vi "Waveform Gen.vi"(9 "Inputs":T1={"Frequency1"=2000.0, "Bit Duration in ms"=0.05, "Frequency2"=4000.0, "Amplitude Scale"=1.0, "Sampling Rate"=50000} {"Frequency2" format="%#_13g"; "Frequency1" format="%#_13g"}, 11 "Message String":string="A") -> (0 "Total Message Duration":dbl=0.4, 1 "Waveform Array":u16[](array[numeric]), 2 "No. of Points":u64=20000, 4 "Actual Message Duration":dbl=0.4, 5 "Waveform Graph":u16[](graph))   [LabVIEW 2021]
uses:
  <vilib>/Analysis/NI_AALPro.lvlib
panel:
  out "length":i32
  out "Array":bool[](array[boolean])
  out "Number of characters possible":dbl
  out "Memory exceeded":bool
  out "size(s)":i32
  out "Bit Stram Indicator":u16
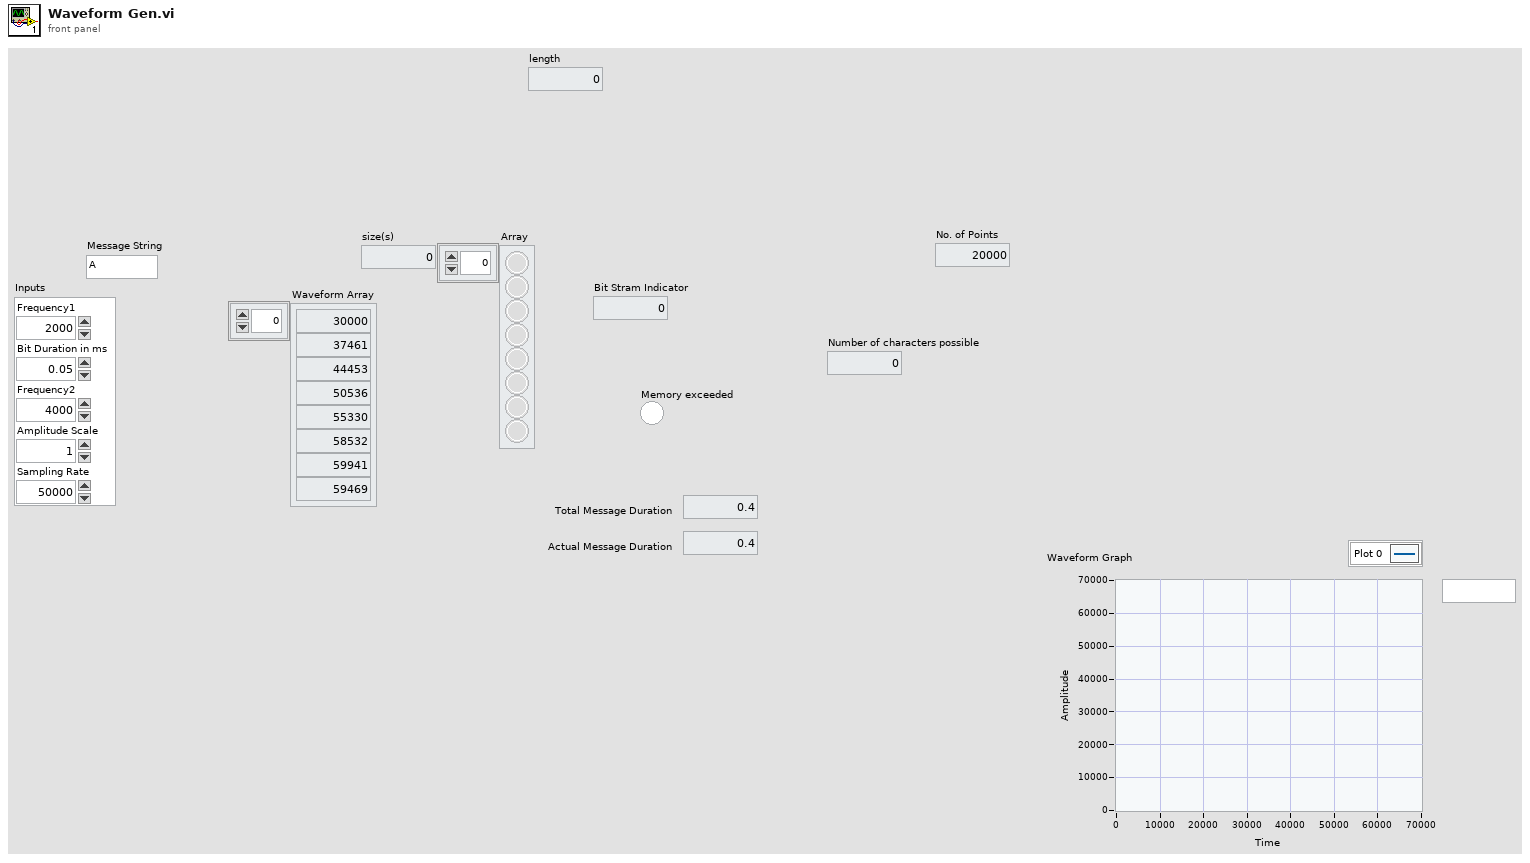
[diagram p1: front panel]
types:
  T1 = cluster{"Frequency1":dbl, "Bit Duration in ms":dbl, "Frequency2":dbl, "Amplitude Scale":dbl, "Sampling Rate":u32}
  T2 = enum16{"sine", "cosine", "triangle", "square", "sawtooth", "increasing ramp", "decreasing ramp"}
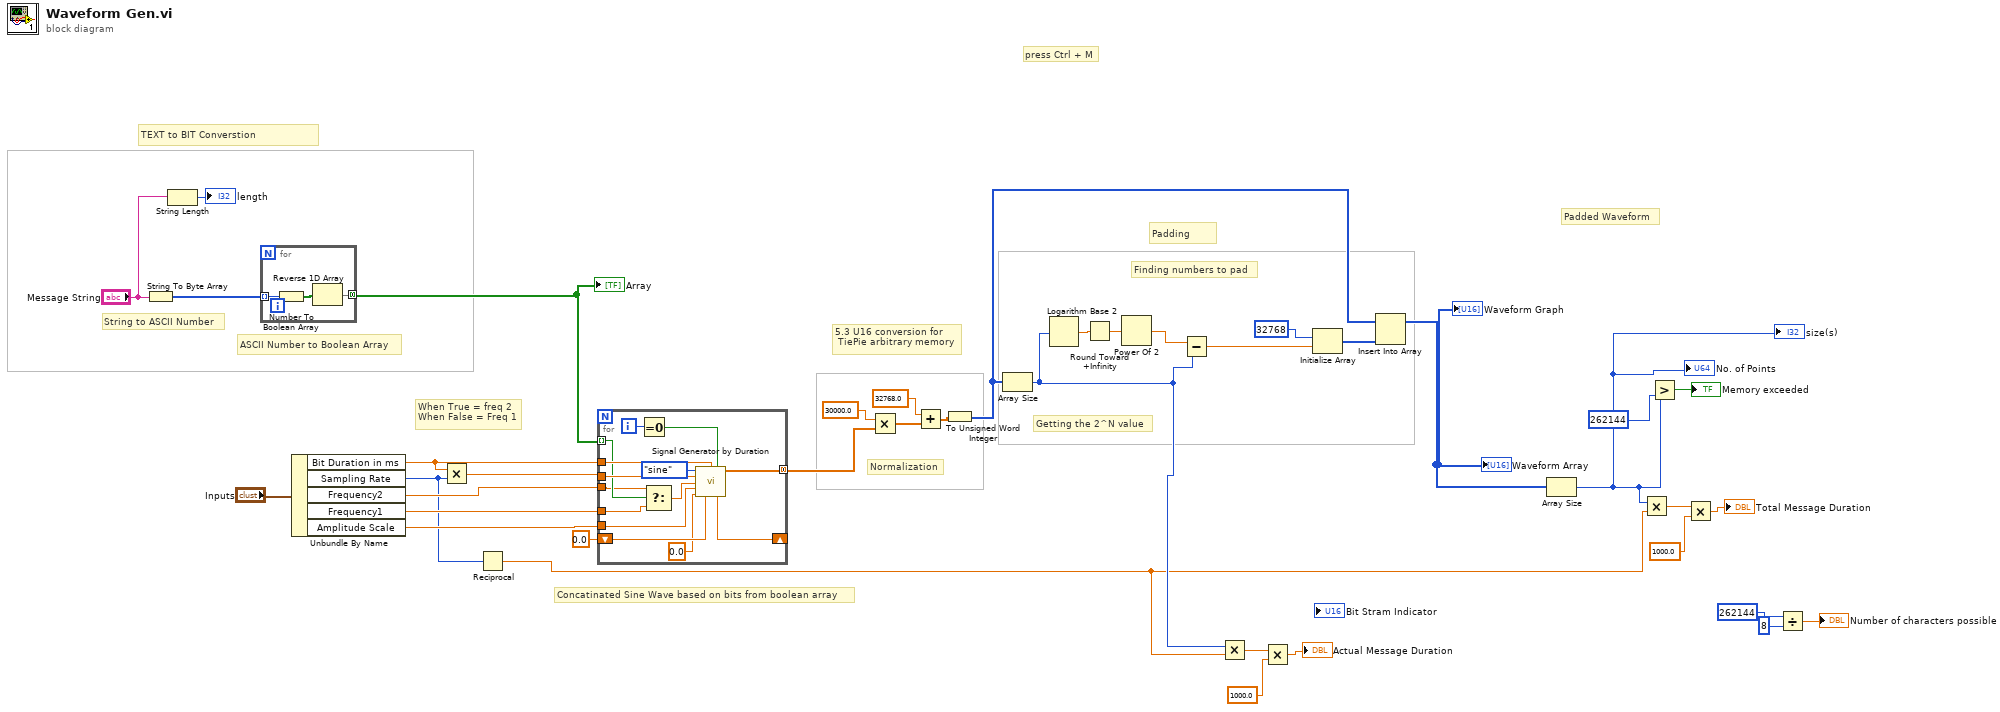
[diagram p0: block diagram]
diagram:
  # "Padding"
  # "5.3 U16 conversion for\n TiePie arbitrary memory"
  # "TEXT to BIT Converstion"
  # "Padded Waveform"
  # "Finding numbers to pad"
  # "Getting the 2^N value"
  # "Normalization"
  # "When True = freq 2\nWhen False = Freq 1"
  # "Concatinated Sine Wave based on bits from boolean array"
  # "ASCII Number to Boolean Array"
  # "String to ASCII Number"
  # "press Ctrl + M"
  n1 = String To Byte Array(string="Message String") -> (unsigned byte array=w39:u8[])
  n2 = String Length(string="Message String") -> (length=→"length":i32)
  n3 = for {
    tunnel: w39 -> [w42] mode=indexing
    tunnel: [w40] -> w38 mode=concatenating
    n4 = Number To Boolean Array(number=w42) -> (Boolean array=w41:bool[])
    n5 = Reverse 1D Array(array=w41) -> (reversed array=w40:bool[])
  }
  "Array" <- w38
  n6 = Unbundle By Name("Inputs") -> ("Bit Duration in ms"=w36:dbl, "Sampling Rate"=w30:u32, "Frequency2"=w34:dbl, "Frequency1"=w33:dbl, "Amplitude Scale"=w31:dbl)
  n7 = Multiply(x=w36, y=w30) -> (x*y=w35:dbl)
  n8 = Reciprocal(x=w30) -> (1/x=w6:dbl)
  n9 = for {
    tunnel: w38 -> [w51] mode=indexing
    tunnel: w36 -> [w54]
    tunnel: w35 -> [w53]
    tunnel: w34 -> [w50]
    tunnel: w33 -> [w49]
    shift-right: [w48] -> _
    shift-left: 0.0 ("phase out") -> [w47]
    tunnel: w31 -> [w44]
    tunnel: [w45] -> w25 mode=concatenating
    i -> [w56]
    n10 = Equal To 0?(x=w56) -> (x = 0?=w55:bool)
    n11 = Select(t=w50, s=w51, f=w49) -> (s? t:f=w52:dbl)
    n12 = call <vilib>:"Signal Generator by Duration.vi"("signal type"=T2."sine", "duration"=w54, "reset phase"=w55, "# of samples"=w53, "frequency"=w52, "amplitude"=w44, "dc offset"=0.0, "phase in"=w47) -> ("signal"=w45:dbl[], "phase out"=w48:dbl)  [unwired: 4 in, 2 out]
  }
  n13 = Multiply(x=30000.0 ("dc offset"), y=w25) -> (x*y=w29:dbl[])
  n14 = Add(x=32768.0 ("dc offset"), y=w29) -> (x+y=w23:dbl[])
  n15 = To Unsigned Word Integer(number=w23) -> (unsigned 16bit integer=w18:u16[])
  n16 = Array Size(array=w18) -> (size(s)=w7:i32)
  n17 = Logarithm Base 2(1:w7) -> (0:w28:dbl)
  n18 = Round Toward +Infinity(x=w28) -> (ceil(x): smallest int >= x=w26:dbl)
  n19 = Power Of 2(x=w26) -> (2^x=w21:dbl)
  n20 = Subtract(x=w21, y=w7) -> (x-y=w20:dbl)
  n21 = Multiply(x=w7, y=w6) -> (x*y=w8:dbl)
  n22 = Multiply(x=w8, y=1000.0) -> (x*y=→"Actual Message Duration":dbl)
  n23 = Initialize Array(u16 32768 ("dc offset"), w20) -> (w17:u16[])
  n24 = Insert Into Array(array=w18, new element=w17) -> (w2:u16[])  [unwired: 1 in]
  "Waveform Array" <- w2
  "Waveform Graph" <- w2
  n25 = Array Size(array=w2) -> (size(s)=w1:i32)
  "No. of Points" <- w1
  "size(s)" <- w1
  n26 = Multiply(x=w1, y=w6) -> (x*y=w27:dbl)
  n27 = Greater?(x=w1, y=262144) -> (0:→"Memory exceeded":bool)
  n28 = Multiply(x=w27, y=1000.0) -> (x*y=→"Total Message Duration":dbl)
  n29 = Divide(x=262144, y=8) -> (x/y=→"Number of characters possible":dbl)
